vi "CalcStability.vi"(8 "error in (no error)":errorcluster, 11 "Control-Client in":refnum<class "Control-Client.lvclass">) -> (0 "error out":errorcluster, 2 "stability":T1(graph), 3 "Control-Client out":refnum<class "Control-Client.lvclass">)   [LabVIEW 2015, in "Control-Client.lvclass"]
uses:
  Control-Client.lvclass
  Experiments/Experiment.lvclass
  <vilib>/Analysis/NI_AALBase.lvlib
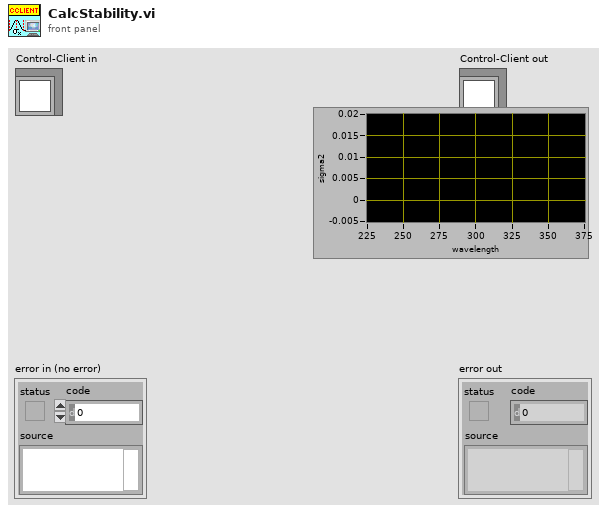
[diagram p1: front panel]
types:
  T1 = cluster{"wavelengths":dbl[], "wavelengths":dbl[]}[]
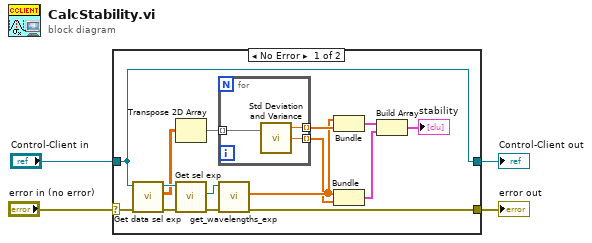
[diagram p0: block diagram]
diagram:
  n1 = case shown="No Error" "error in (no error)" {
    selector: "error in (no error)" -> [w18 w24]
    tunnel: [w13 w24] -> w3
    tunnel: [w19 w23] -> w1
    tunnel: "Control-Client in" -> [w19 w23]
    frame No Error {
      n2 = call "Get data sel exp.vi"("error in (no error)"=w18, "Control-Client in"=w19) -> ("error out"=w16:errorcluster, "Data"=w6:sgl[][], "Control-Client out"=w17:refnum<class "Control-Client.lvclass">)  [unwired: 7 in]
      n3 = Transpose 2D Array(2D array=w6) -> (transposed array=w5:sgl[][])
      n4 = call "Get sel exp.vi"("error in (no error)"=w16, "Control-Client in"=w17) -> ("error out"=w15:errorcluster, "Sel experiment"=w14:refnum<class "Experiment.lvclass">)  [unwired: 7 in, 1 out]
      n5 = for {
        tunnel: w5 -> [w22] mode=indexing
        tunnel: [w21] -> w8 mode=indexing
        tunnel: [w20] -> w10 mode=indexing
        n6 = call <vilib>:"Std Deviation and Variance.vi"("X"=w22) -> ("mean"=w20:dbl, "standard deviation"=w21:dbl)  [unwired: 1 in, 1 out]
      }
      n7 = call "get_wavelengths_exp.vi"("error in (no error)"=w15, "Experiment.lvclass in"=w14) -> ("error out"=w13:errorcluster, "wavelengths"=w9:dbl[])  [unwired: 7 in, 1 out]
      n8 = Bundle("wavelengths"=w9, w10) -> (w12:cluster{"wavelengths":dbl[], dbl[]})  [unwired: 1 in]
      n9 = Bundle("wavelengths"=w9, w8) -> (w7:cluster{"wavelengths":dbl[], dbl[]})  [unwired: 1 in]
      n10 = Build Array(w12, w7) -> (→"stability":cluster{"wavelengths":dbl[], dbl[]}[])
    }
    frame Error {
    }
  }
  "error out" <- w3
  "Control-Client out" <- w1
